vi "ESC Sensor (for testing only - probably does not work).vi"() -> ()   [LabVIEW 2016]
panel:
  in  "threshold":dbl
  out "above threshold (\"radar detected\")":bool
  out "concatenated string":string
  in  "file path (use dialog)":path
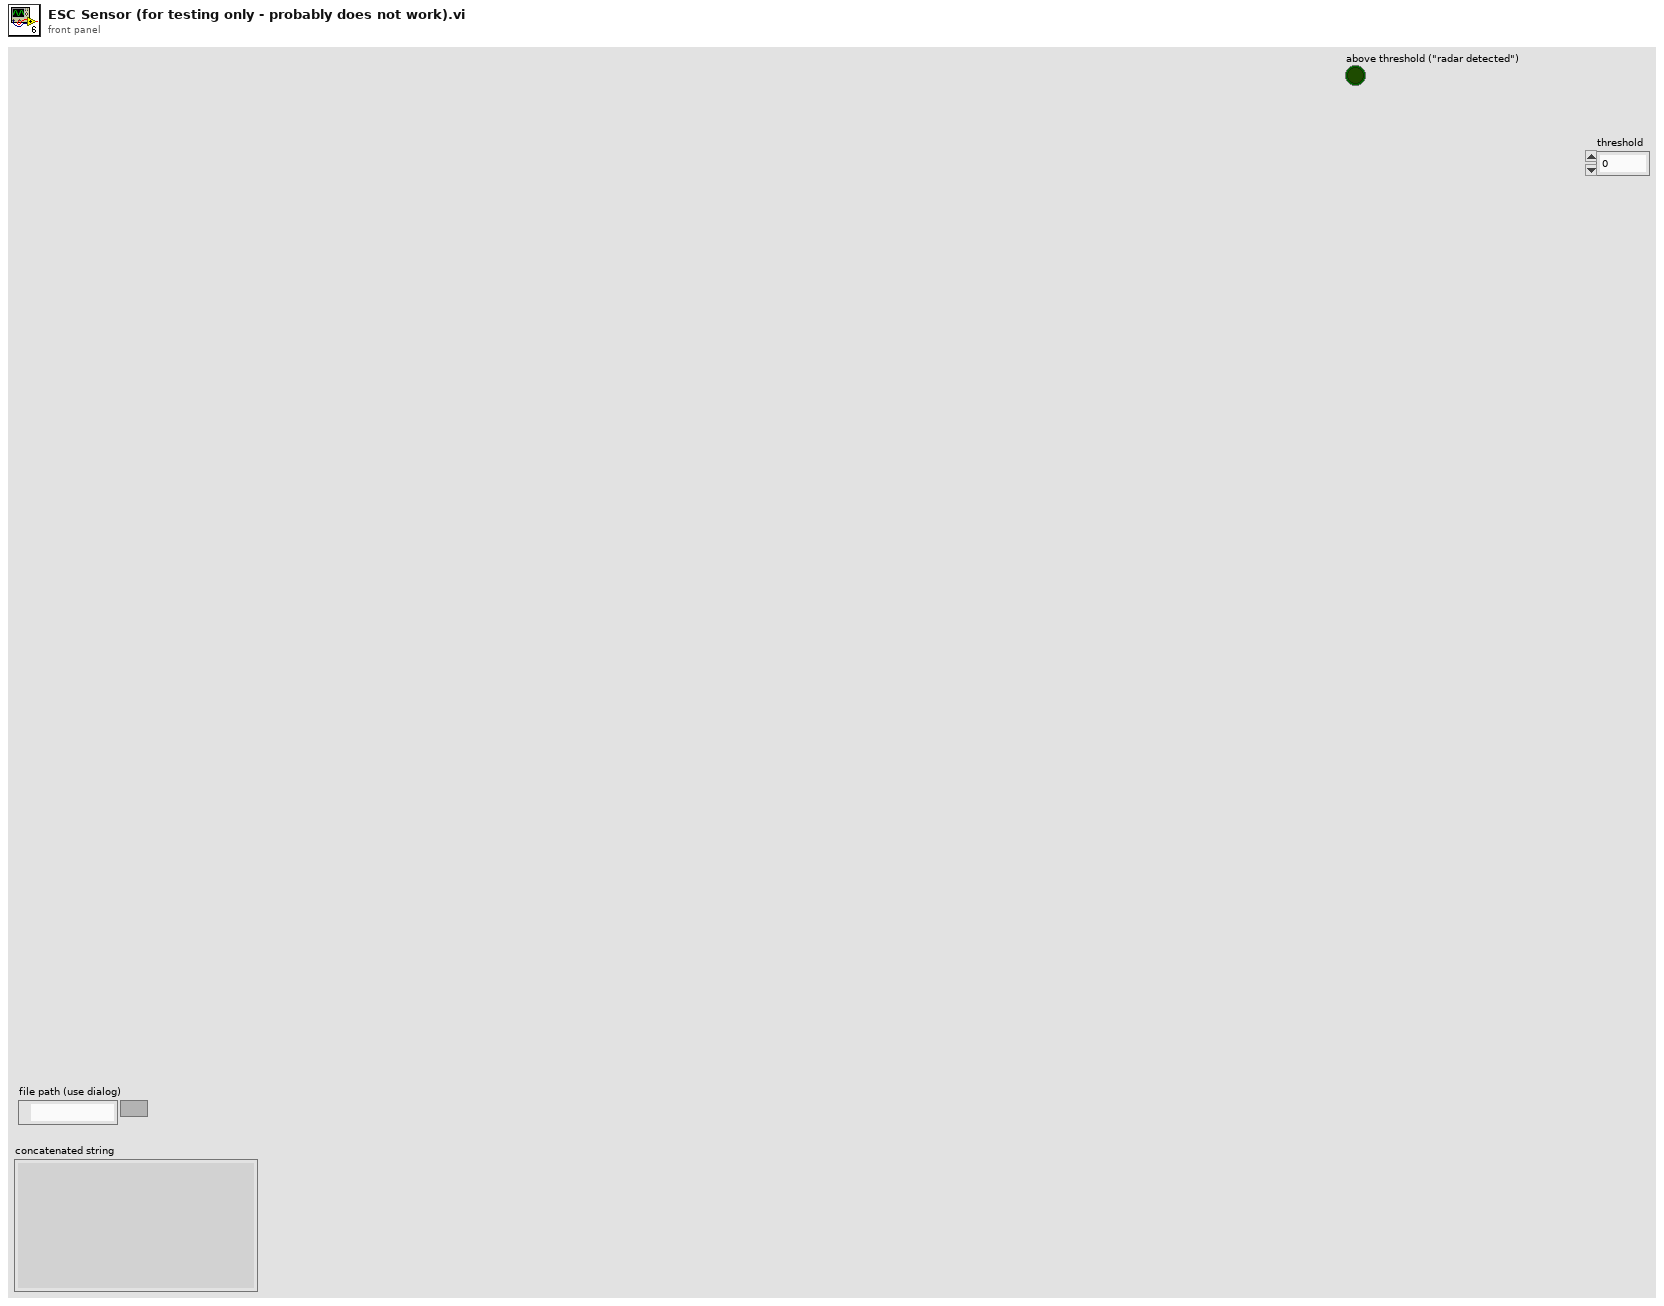
[diagram p1: front panel]
types:
  T1 = enum16{"open", "replace", "create", "open or create", "replace or create", "replace or create with confirmation"}
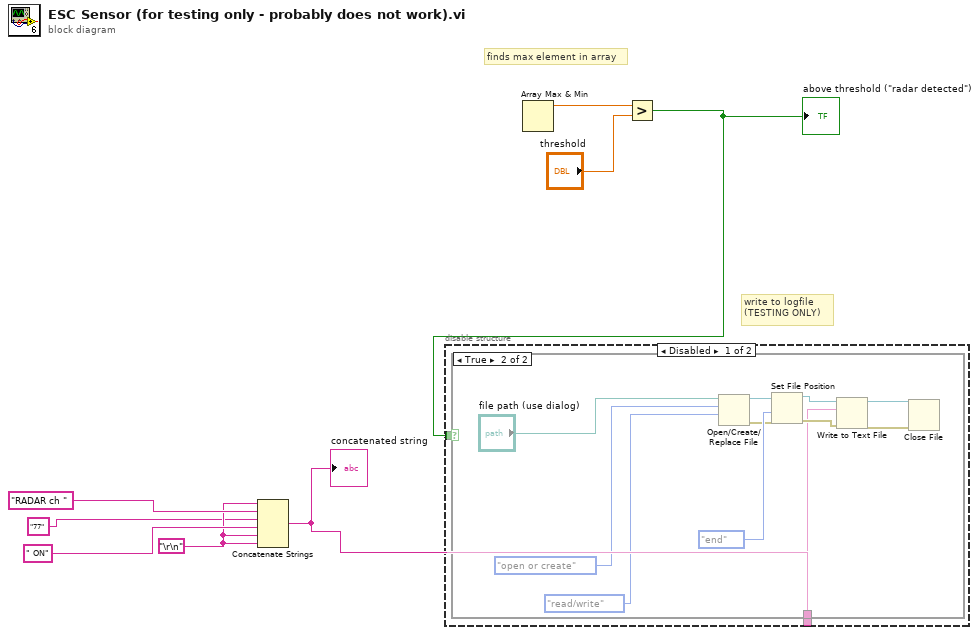
[diagram p0: block diagram]
diagram:
  w3 = "\r\n"
  # "write to logfile\n(TESTING ONLY)"
  # "finds max element in array"
  n1 = Concatenate Strings(w3, "RADAR ch " ("string"), "77" ("string"), " ON" ("string"), w3, w3) -> (w1:string)
  "concatenated string" <- w1
  n2 = Array Max & Min() -> (max value=w8:dbl)  [unwired: 1 in, 3 out]
  n3 = Greater?(x=w8, y="threshold") -> (0:w6:bool)
  "above threshold (\"radar detected\")" <- w6
  n4 = disable-structure shown="Disabled" {
    disable-tunnel: w6 -> [w10 _]
    disable-tunnel: w1 -> [w9 _]
    frame Disabled {
      n5 = case shown="True" w10 {
        tunnel: w9 -> [_ w11]
        frame False {
        }
        frame True {
          n6 = Open/Create/Replace File(file path (use dialog)="file path (use dialog)", operation (0:open)=T1."open or create", access (0:read/write)=enum16{"read/write", "read-only", "write-only"}."read/write") -> (refnum out=w15:refnum<file>, error out=w13:errorcluster)  [unwired: 3 in, 1 out]
          n7 = Set File Position(refnum=w15, from (0:start)=enum16{"start", "end", "current"}."end", error in=w13) -> (refnum out=w14:refnum<file>, error out=w12:errorcluster)  [unwired: 1 in]
          n8 = Write to Text File(file (use dialog)=w14, text=w11, error in=w12) -> (refnum out=w18:refnum<file>, error out=w17:errorcluster)  [unwired: 1 in, 1 out]
          n9 = Close File(refnum=w18, error in=w17) -> ()  [unwired: 2 out]
        }
      }
    }
    frame Enabled {
    }
  }
